vi "Evaluate Insertion Request.vi"(10 "Insertion Request Time":timestamp, 11 "ProtectedSubpanel":refnum<class "ProtectedSubpanel.lvclass">) -> (3 "Perform Insertion?":bool)   [LabVIEW 2017, in "IViewable.lvlib" / "ProtectedSubpanel.lvclass"]
uses:
  ProtectedSubpanel.lvclass
  ProtectedSubpanel.lvclass/ProtectedSubpanel.ctl
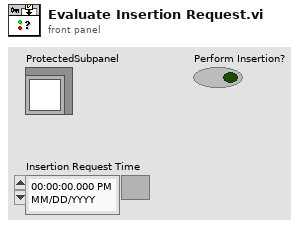
[diagram p1: front panel]
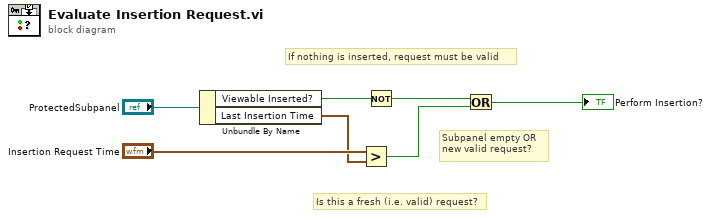
[diagram p0: block diagram]
diagram:
  # "If nothing is inserted, request must be valid"
  # "Subpanel empty OR\nnew valid request?"
  # "Is this a fresh (i.e. valid) request?"
  n1 = Unbundle By Name("ProtectedSubpanel") -> ("Viewable Inserted?"=w2:bool, "Last Insertion Time"=w1:timestamp)
  n2 = Greater?(x="Insertion Request Time", y=w1) -> (0:w4:bool)
  n3 = Not(x=w2) -> (.not. x?=w3:bool)
  n4 = Or(x=w3, y=w4) -> (x .or. y?=→"Perform Insertion?":bool)
